vi "Write Data.vi"(8 "error in (no error)":errorcluster, 9 "Publication Time":timestamp, 10 "Value":variant, 11 "ConfigurationFileBinding In":refnum<class "ConfigurationFileBinding.lvclass">) -> (0 "error out":errorcluster, 3 "ConfigurationFileBinding Out":refnum<class "ConfigurationFileBinding.lvclass">)   [LabVIEW 2017, in "Transport.lvlib" / "ConfigurationFileBinding.lvclass"]
doc: "<License>\nCopyright © 2017 Composed Systems, LLC | All rights reserved\nwww.composed.io\n\nAuthor: Ethan Stern <ethan.stern@composed.io>\n\nThis software is provided \"AS IS\" WITHOUT WARRANTIES, either express or implied, AND IS FOR EDUCATIONAL PURPOSES ONLY.\n</License>"
uses:
  ConfigurationFileBinding.lvclass
  ConfigurationFileBinding.lvclass/ConfigurationFileBinding.ctl
  <vilib>/Utility/config.llb/Write Key (Path).vi
  <vilib>/Utility/config.llb/Write Key (String).vi
  <vilib>/Utility/config.llb/Write Key (Boolean).vi
  <vilib>/Utility/config.llb/Write Key (Double).vi
  <vilib>/Utility/config.llb/Write Key (U32).vi
  <vilib>/Utility/config.llb/Write Key (I32).vi
  <vilib>/Utility/error.llb/Error Cluster From Error Code.vi
  <vilib>/ErrorRing/Error Ring.xnode
  <vilib>/Utility/Data Type/NI_Data Type.lvlib
  <vilib>/Utility/config.llb/NI_LVConfig.lvlib
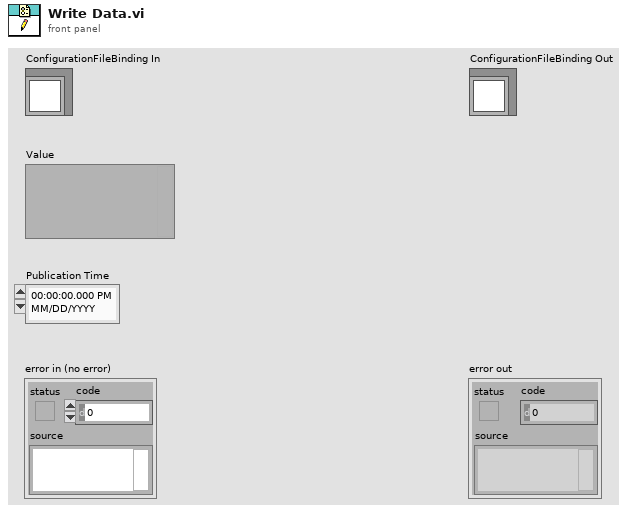
[diagram p1: front panel]
types:
  T1 = typedef "NI_LVConfig.lvlib/Config Data RefNum.ctl" = refnum<k1>
  T2 = typedef "NI_Data Type.lvlib/Data Type.ctl" = enum8{"Invalid Type", "Void", "I8", "I16", "I32", "I64", "U8", "U16", "U32", "U64", "Single Float", "Double Float", "Extended Float", "Single Complex", "Double Complex", "Extended Complex", "Enum U8", "Enum U16", "Enum U32", "Enum U64", "Single Float With Unit", "Double Float With Unit", "Extended Float With Unit", "Single Complex with Unit", "Double Complex with Unit", "Extended Complex with Unit", "Boolean", "String", "Path", "Picture", "Tag", "Array", "Cluster", "Variant", "LV Variant", "Waveform", "Timestamp", "Digital Waveform", "Digital Data", "ExpressData", "Refnum", "External Data", "VI", "Poly VI", "LabVIEW Class Instance", "Fixed Point"}
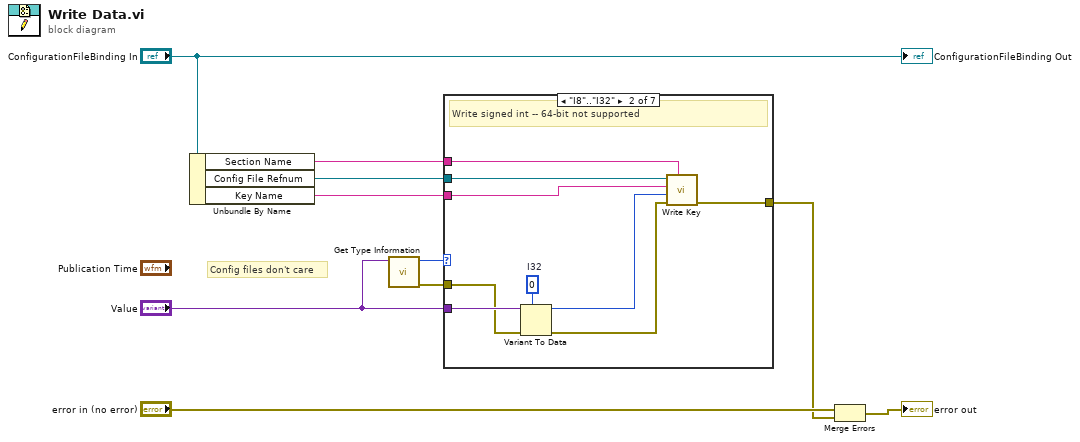
[diagram p0: block diagram]
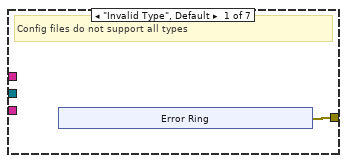
[diagram p2: hidden frame]
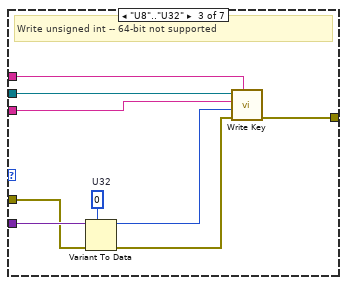
[diagram p3: hidden frame]
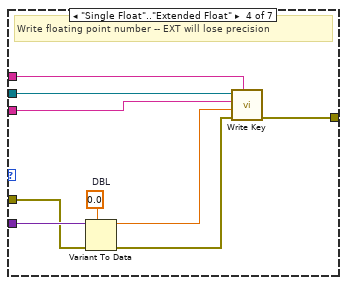
[diagram p4: hidden frame]
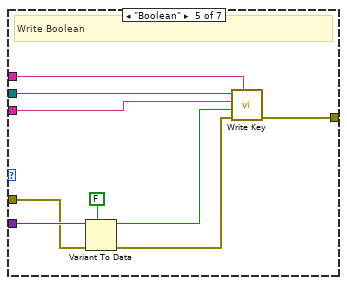
[diagram p5: hidden frame]
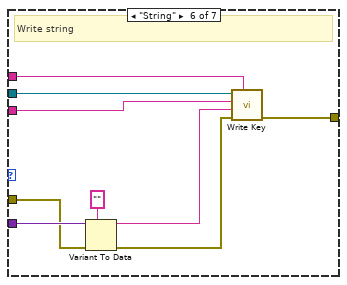
[diagram p6: hidden frame]
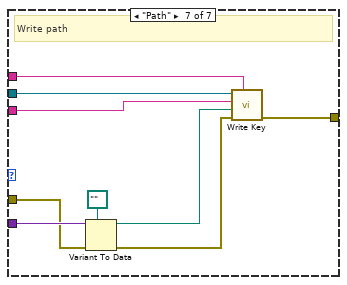
[diagram p7: hidden frame]
diagram:
  # "Config files don't care"
  n1 = Unbundle By Name("ConfigurationFileBinding In") -> ("Section Name"=w4:string, "Config File Refnum"=w5:T1, "Key Name"=w3:string)
  n2 = call <vilib>:"Get Type Information.vi"("Variant"="Value") -> ("error out"=w1:errorcluster, "Type"=w2:T2)  [unwired: 6 in, 3 out]
  n3 = case shown="\"I8\"..\"I32\"" w2 {
    tunnel: [w11 w24 w33 w42 w51 w60 w69] -> w7
    tunnel: w3 -> [_ w21 w30 w39 w48 w57 w66]
    tunnel: "Value" -> [_ w20 w29 w38 w47 w56 w65]
    tunnel: w5 -> [_ w22 w31 w40 w49 w58 w67]
    tunnel: w1 -> [_ w19 w28 w37 w46 w55 w64]
    tunnel: w4 -> [_ w18 w27 w36 w45 w54 w63]
    frame "Invalid Type", Default {
      # "Config files do not support all types"
      n4 = xnode "Error Ring"() -> ("error out"=w11:errorcluster)
    }
    frame "I8".."I32" {
      w23 = 0  # I32
      # "Write signed int -- 64-bit not supported"
      n5 = Variant To Data(error in=w19, type=w23, Variant=w20) -> (data=w16:i32, error out=w17:errorcluster)
      n6 = call-poly <vilib>:"Write Key.vi"("section"=w18, "error in (no error)"=w17, "value"=w16, "key"=w21, "refnum"=w22) -> ("error out"=w24:errorcluster)  [unwired: 4 in, 2 out]
    }
    frame "U8".."U32" {
      w32 = u32 0  # U32
      # "Write unsigned int -- 64-bit not supported"
      n7 = Variant To Data(error in=w28, type=w32, Variant=w29) -> (data=w25:u32, error out=w26:errorcluster)
      n8 = call-poly <vilib>:"Write Key.vi"("section"=w27, "error in (no error)"=w26, "value"=w25, "key"=w30, "refnum"=w31) -> ("error out"=w33:errorcluster)  [unwired: 4 in, 2 out]
    }
    frame "Single Float".."Extended Float" {
      w41 = 0.0  # DBL
      # "Write floating point number -- EXT will lose precision"
      n9 = Variant To Data(error in=w37, type=w41, Variant=w38) -> (data=w34:dbl, error out=w35:errorcluster)
      n10 = call-poly <vilib>:"Write Key.vi"("section"=w36, "error in (no error)"=w35, "value"=w34, "key"=w39, "refnum"=w40) -> ("error out"=w42:errorcluster)  [unwired: 4 in, 2 out]
    }
    frame "Boolean" {
      # "Write Boolean"
      n11 = Variant To Data(error in=w46, type=FALSE, Variant=w47) -> (data=w43:bool, error out=w44:errorcluster)
      n12 = call-poly <vilib>:"Write Key.vi"("section"=w45, "error in (no error)"=w44, "value"=w43, "key"=w48, "refnum"=w49) -> ("error out"=w51:errorcluster)  [unwired: 4 in, 2 out]
    }
    frame "String" {
      # "Write string"
      n13 = Variant To Data(error in=w55, type="", Variant=w56) -> (data=w52:string, error out=w53:errorcluster)
      n14 = call-poly <vilib>:"Write Key.vi"("section"=w54, "error in (no error)"=w53, "value"=w52, "key"=w57, "refnum"=w58) -> ("error out"=w60:errorcluster)  [unwired: 4 in, 2 out]
    }
    frame "Path" {
      # "Write path"
      n15 = Variant To Data(error in=w64, type=path "", Variant=w65) -> (data=w61:path, error out=w62:errorcluster)
      n16 = call-poly <vilib>:"Write Key.vi"("section"=w63, "error in (no error)"=w62, "value"=w61, "key"=w66, "refnum"=w67) -> ("error out"=w69:errorcluster)  [unwired: 4 in, 2 out]
    }
  }
  n17 = Merge Errors("error in (no error)", w7) -> (→"error out":errorcluster)
  "ConfigurationFileBinding Out" <- "ConfigurationFileBinding In"
